vi "Generate EPICS server URL.vi"(11 "machine":string="localhost") -> (3 "EPICS server URL":string)   [LabVIEW 2011]
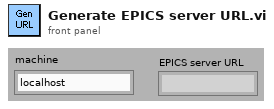
[diagram p1: front panel]
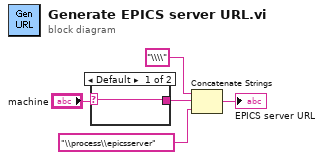
[diagram p0: block diagram]
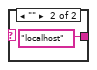
[diagram p2: hidden frame]
diagram:
  n1 = case shown="Default" "machine" {
    selector: "machine" -> [w6 _]
    tunnel: [w6 "localhost"] -> w1
    frame Default {
    }
    frame "" {
    }
  }
  n2 = Concatenate Strings("\\\\" ("string"), w1, "\\process\\epicsserver" ("string")) -> (→"EPICS server URL":string)
